vi "test Triggered Acyclic Frame.vi"(8 "error in":errorcluster, 11 "Loopback in":refnum<class "Loopback.lvclass">) -> (0 "error out":errorcluster, 3 "Loopback out":refnum<class "Loopback.lvclass">)   [LabVIEW 2020, in "Loopback.lvclass"]
uses:
  Loopback.lvclass
  C:/Users/nitest/Desktop/Git 2020/niveristand-custom-device-testing-tools/VeriStandTestCase/VeriStandTestCase.lvclass
  <vilib>/NI VeriStand/Execution/Workspace/NI VeriStand - Set Single Channel Value.vi
  niveristand-custom-device-testing-tools/VeriStandTestUtilities/VeriStandTestUtilities.lvlib
  <vilib>/NI VeriStand/Execution/Workspace/NI_VS Workspace ExecutionAPI.lvlib
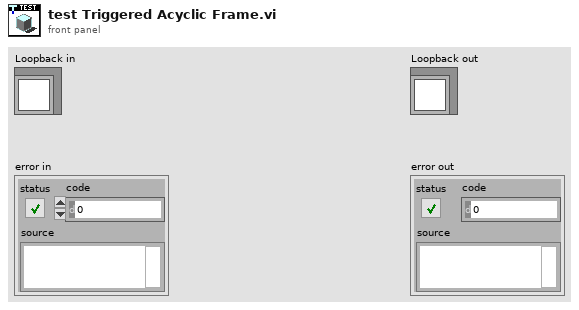
[diagram p1: front panel]
types:
  T1 = typedef "NI_VS Workspace ExecutionAPI.lvlib/WorkspaceAPI.ctl" = refnum<k24>
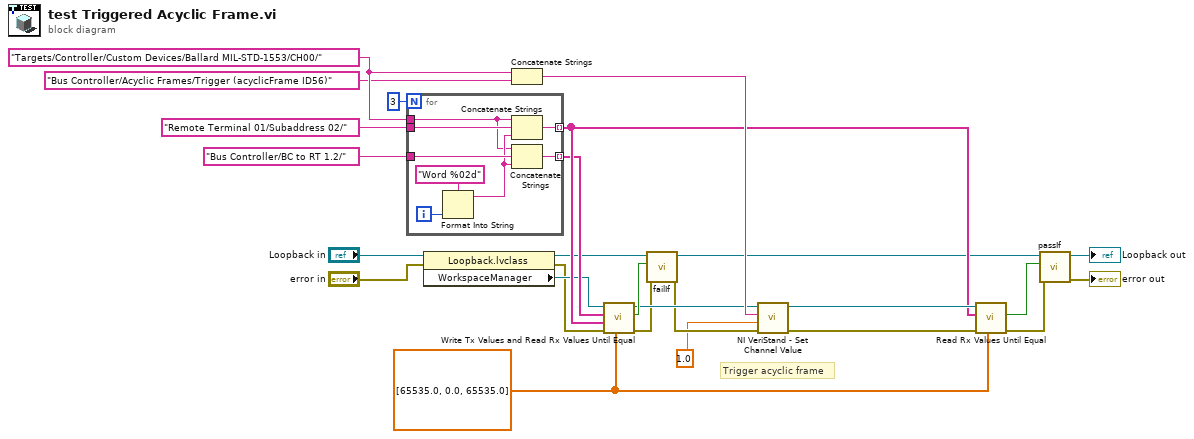
[diagram p0: block diagram]
diagram:
  w26 = "Targets/Controller/Custom Devices/Ballard MIL-STD-1553/CH00/" ("base name for channel aliases")
  w21 = dbl[] [65535.0, 0.0, 65535.0]
  # "Trigger acyclic frame"
  n1 = for {
    N: 3 -> [_]
    tunnel: "Bus Controller/BC to RT 1.2/" ("Channel") -> [w33]
    tunnel: [w34] -> w12 mode=indexing
    tunnel: "Remote Terminal 01/Subaddress 02/" ("Channel") -> [w32]
    tunnel: [w31] -> w14 mode=indexing
    tunnel: w26 -> [w27]
    i -> [w30]
    n2 = Format Into String(format string="Word %02d", w30) -> (resulting string=w29:string)  [unwired: 2 in, 1 out]
    n3 = Concatenate Strings(w27, w32, w29) -> (w31:string)
    n4 = Concatenate Strings(w27, w33, w29) -> (w34:string)
  }
  n5 = property class="Loopback.lvclass"(reference="Loopback in", error in="error in") -> (reference out=w1:refnum<class "Loopback.lvclass">, error out=w2:errorcluster, "WorkspaceManager"=w5:T1)
  n6 = Concatenate Strings(w26, "Bus Controller/Acyclic Frames/Trigger (acyclicFrame ID56)") -> (w23:string)
  n7 = call "Write Tx Values and Read Rx Values Until Equal.vi"("Tx values"=w21, "error in"=w2, "Rx aliases"=w14, "Tx aliases"=w12, "workspace manager in"=w5) -> ("error out"=w13:errorcluster, "values equal"=w20:bool, "workspace manager out"=w16:T1)  [unwired: 4 in]
  n8 = call-dynamic "failIf.vi"("error in (no error)"=w13, "fail"=w20, "TestCase in"=w1) -> ("error out"=w10:errorcluster, "TestCase out"=w11:refnum<class "Loopback.lvclass">)  [unwired: 7 in]
  n9 = call-poly <vilib>:"NI VeriStand - Set Channel Value.vi"("error in (no error)"=w10, "Value"=1.0, "Channel"=w23, "WorkspaceManager in"=w16) -> ("error out"=w19:errorcluster, "WorkspaceManager out"=w18:T1)  [unwired: 6 in]
  n10 = call "Read Rx Values Until Equal.vi"("expected values"=w21, "error in"=w19, "Rx aliases"=w14, "workspace manager in"=w18) -> ("error out"=w17:errorcluster, "values equal expected"=w15:bool)  [unwired: 5 in, 1 out]
  n11 = call-dynamic "passIf.vi"("error in (no error)"=w17, "pass"=w15, "TestCase in"=w11) -> ("error out"=→"error out":errorcluster, "TestCase out"=→"Loopback out":refnum<class "Loopback.lvclass">)  [unwired: 7 in]
